vi "Oscilloscope_Dual_MohammadVersion.vi"() -> ()   [LabVIEW 2024]
uses:
  <vilib>/DAQmx/read.llb/DAQmx Read (Analog 1D Wfm NChan NSamp).vi
  <vilib>/DAQmx/create/channels.llb/DAQmx Create Channel (AI-Voltage-Basic).vi
  <vilib>/DAQmx/configure/timing.llb/DAQmx Timing (Sample Clock).vi
  <vilib>/DAQmx/configure/trigger.llb/DAQmx Start Trigger (Analog Edge).vi
  <vilib>/DAQmx/miscellaneous.llb/DAQmx Fill In Error Info.vi
panel:
  in  "stop":bool
  in  "Trigger source":string
  in  "File Logging":bool
  in  "Trigger Mode":bool
  in  "level":dbl format="%0.2f"
  out "right 2":dynamicdata(graph)=[{"t0"=timestamp(3806599236.6321588 s since 1904-01-01), "dt"=4.999999999999579e-07, "Y"=array[202167 elements], "attributes"=variant("NI_ChannelName"=variant(string "cDAQ2Mod1/ai1"), "NI_UnitDescription"=variant(string "Volts"))}]
  out "left 2":dynamicdata(graph)=[{"t0"=timestamp(3806599236.6321588 s since 1904-01-01), "dt"=4.999999999999579e-07, "Y"=array[202167 elements], "attributes"=variant("NI_ChannelName"=variant(string "cDAQ2Mod1/ai0"), "NI_UnitDescription"=variant(string "Volts"))}]
  in  "stop Acquisition":bool
  in  "File Name":string
  in  "Folder to save file to":path=path "A:/Source Localization/Material Evaluation paper/Dataset/Microphone Characterization/Clean Source"
  in  "physical channels":tag="cDAQ2Mod1/ai0, cDAQ2Mod1/ai3"
  in  "Sample Rate":dbl=200000.0 format="%0.2f"
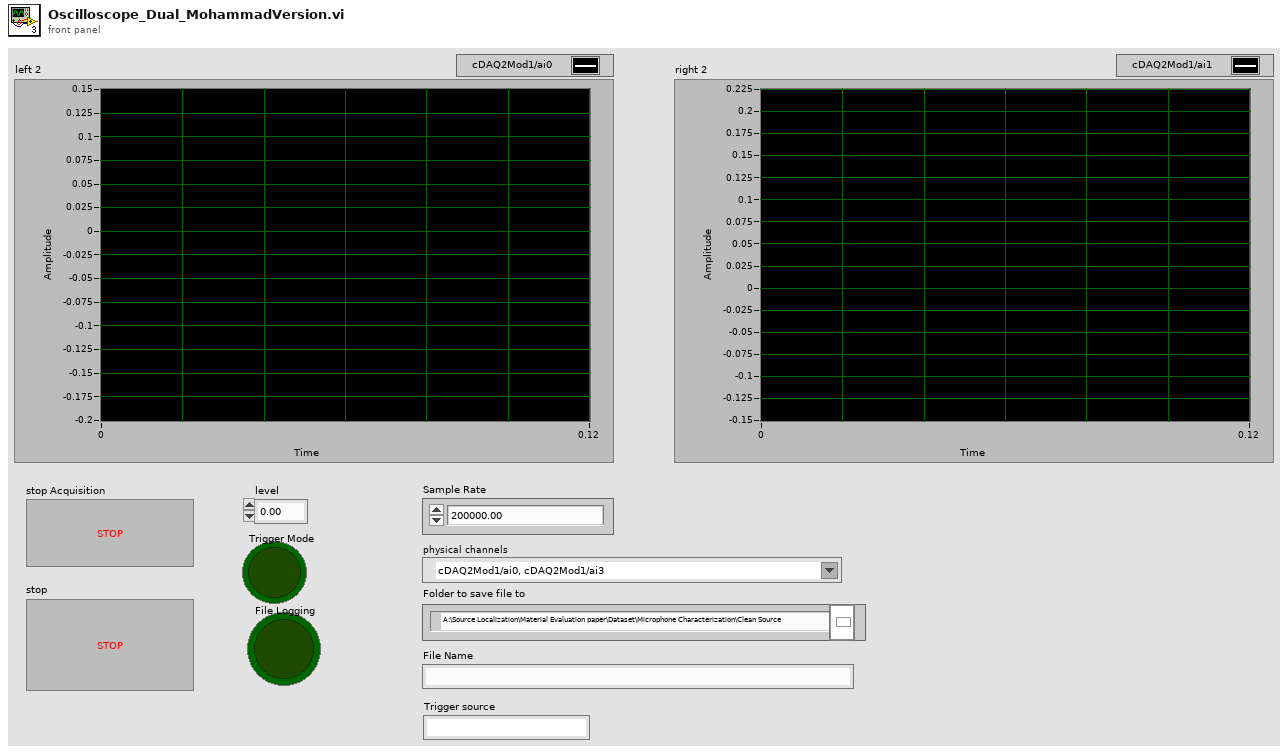
[diagram p1: front panel]
types:
  T1 = enum16{"open", "open or create", "create or replace", "create", "open (read-only)"}
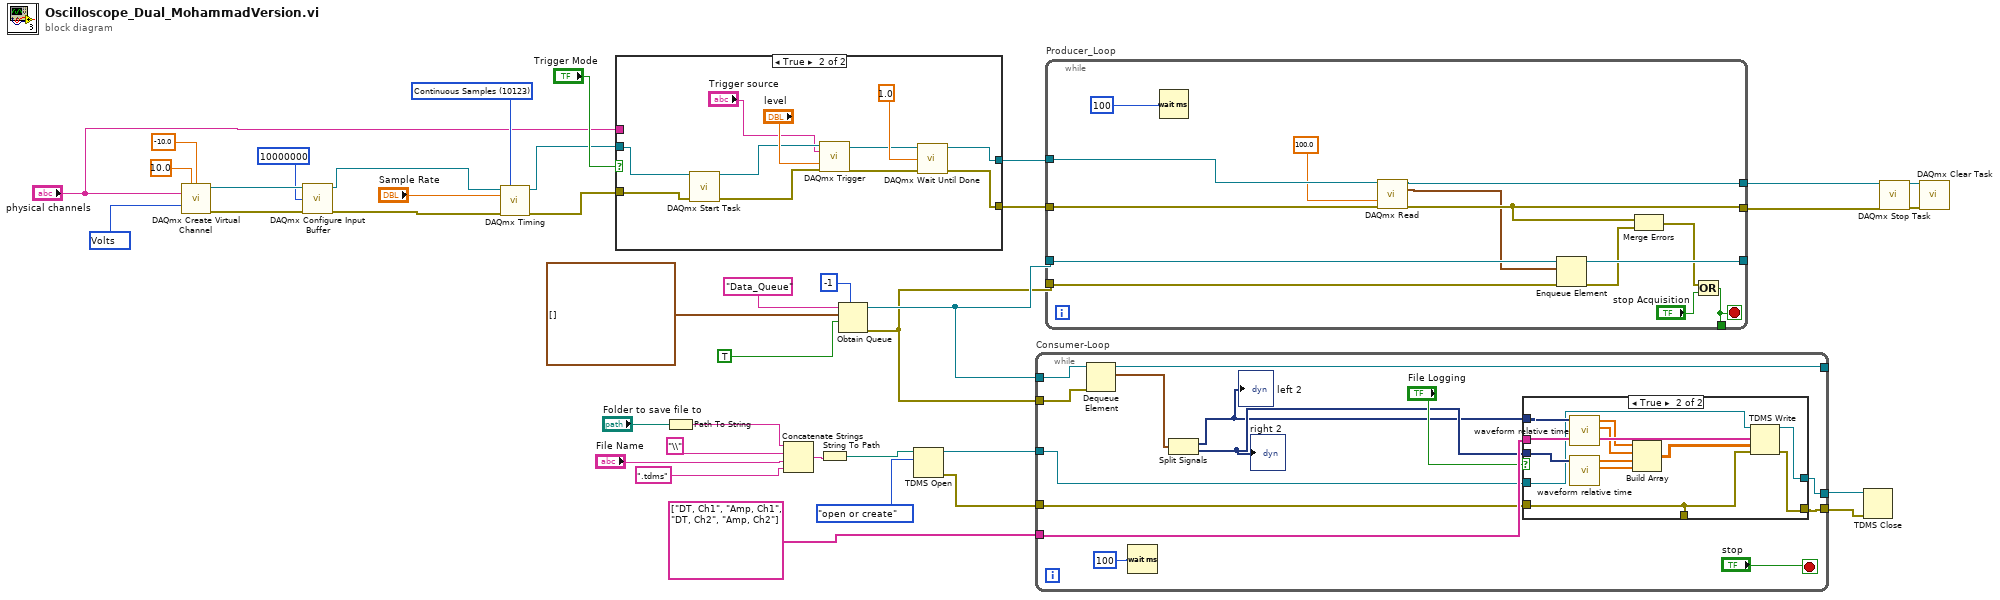
[diagram p0: block diagram]
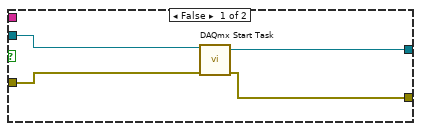
[diagram p2: hidden frame]
diagram:
  w10 = 10348 items=["Volts"=10348, "From Custom Scale"=10065] ("units")
  w34 = 10123 items=["Finite Samples"=10178, "Continuous Samples"=10123, "Hardware Timed Single Point"=12522] ("sample mode")
  n1 = call-poly <vilib>:"DAQmx Create Virtual Channel.vi"("maximum value"=10.0, "minimum value"=-10.0, "physical channels"="physical channels", "units"=w10) -> ("task out"=w39:refnum<k21>, "error out"=w38:errorcluster)  [unwired: 10 in]
  n2 = call <vilib>:"DAQmx Configure Input Buffer.vi"("task/channels in"=w39, "buffer size (in samples per channel)"=u32 10000000, "error in"=w38) -> ("task out"=w36:refnum<k21>, "error out"=w35:errorcluster)  [unwired: 11 in]
  n3 = call-poly <vilib>:"DAQmx Timing.vi"("task/channels in"=w36, "sample mode"=w34, "rate"="Sample Rate", "error in"=w35) -> ("task out"=w7:refnum<k21>, "error out"=w8:errorcluster)  [unwired: 10 in]
  n4 = case shown="True" "Trigger Mode" {
    tunnel: w8 -> [w41 w45]
    tunnel: w7 -> [w42 w46]
    tunnel: [w43 w50] -> w4
    tunnel: [w40 w49] -> w3
    tunnel: "physical channels" -> [_ _]
    frame False {
      n5 = call <vilib>:"DAQmx Start Task.vi"("task/channels in"=w42, "error in"=w41) -> ("task out"=w43:refnum<k21>, "error out"=w40:errorcluster)  [unwired: 12 in]
    }
    frame True {
      n6 = call <vilib>:"DAQmx Start Task.vi"("task/channels in"=w46, "error in"=w45) -> ("task out"=w48:refnum<k21>, "error out"=w47:errorcluster)  [unwired: 12 in]
      n7 = call-poly <vilib>:"DAQmx Trigger.vi"("task/channels in"=w48, "source"="Trigger source", "level"="level", "error in"=w47) -> ("task out"=w52:refnum<k21>, "error out"=w51:errorcluster)  [unwired: 10 in]
      n8 = call <vilib>:"DAQmx Wait Until Done.vi"("task/channels in"=w52, "timeout (sec)"=1.0, "error in"=w51) -> ("task out"=w50:refnum<k21>, "error out"=w49:errorcluster)  [unwired: 11 in]
    }
  }
  n9 = Path To String(path="Folder to save file to") -> (string=w29:string)
  n10 = Concatenate Strings(w29, "\\" ("string"), "File Name", ".tdms" ("string")) -> (w28:string)
  n11 = String To Path(string=w28) -> (path=w25:path)
  n12 = Obtain Queue(max queue size (-1, unlimited)=-1, name (unnamed)="Data_Queue", element data type=waveform(dbl)[] [] ("waveform"), create if not found? (T)=TRUE) -> (queue out=w19:refnum<queue>, error out=w15:errorcluster)  [unwired: 1 in, 1 out]
  n13 = TDMS Open(10:T1."open or create" ("operation (0:open)"), 11:w25) -> (0:w18:errorcluster, 3:w1:refnum<k34>)  [unwired: 5 in]
  n14 = while "Consumer-Loop" {
    tunnel: w19 -> [w68]
    tunnel: w18 -> [w62]
    tunnel: w15 -> [w67]
    tunnel: [w66] -> _
    tunnel: string[] ["DT, Ch1", "Amp, Ch1", "DT, Ch2", "Amp, Ch2"] ("channel name(s) in (Untitled)") -> [w65]
    tunnel: [w63] -> w13
    tunnel: [w61] -> w5
    tunnel: w1 -> [w57]
    stop <- "stop" stop-if-true
    n15 = Dequeue Element(queue=w68, error in (no error)=w67) -> (queue out=w66:refnum<queue>, element=w64:waveform(dbl)[])  [unwired: 1 in, 2 out]
    n16 = Wait (ms)(milliseconds to wait=u32 100) -> ()  [unwired: 1 out]
    n17 = Split Signals(w64) -> (w58:dynamicdata, w59:dynamicdata)  [unwired: 2 in]
    "left 2" <- w58
    "right 2" <- w59
    n18 = case shown="True" "File Logging" {
      tunnel: w65 -> [_ w82]
      tunnel: [w69 w81] -> w63
      tunnel: w62 -> [w70 w80]
      tunnel: [w70 w80] -> _
      tunnel: [w70 w79] -> w61
      tunnel: w59 -> [_ w74]
      tunnel: w58 -> [_ w73]
      tunnel: w57 -> [w69 w71]
      frame False {
      }
      frame True {
        n19 = call "waveform relative time.vi"("signal in"=w73) -> ("Y"=w78:dbl[], "Relative Time"=w77:dbl[])  [unwired: 7 in, 2 out]
        n20 = call "waveform relative time.vi"("signal in"=w74) -> ("Y"=w75:dbl[], "Relative Time"=w76:dbl[])  [unwired: 7 in, 2 out]
        n21 = Build Array(w77, w78, w76, w75) -> (w72:dbl[][])
        n22 = TDMS Write(0:w71, 7:w82, 9:w72, 11:w80) -> (4:w81:refnum<k34>, 15:w79:errorcluster)  [unwired: 2 in, 2 out]
      }
    }
  }
  n23 = while "Producer_Loop" {
    tunnel: w4 -> [w94]
    tunnel: w3 -> [w93]
    tunnel: w19 -> [w96]
    tunnel: w15 -> [w95]
    tunnel: [w92] -> _
    tunnel: [w88] -> w17
    tunnel: [w87] -> w16
    tunnel: [w83] -> _
    stop <- w83 stop-if-true
    n24 = Wait (ms)(milliseconds to wait=u32 100) -> ()  [unwired: 1 out]
    n25 = call-poly <vilib>:"DAQmx Read.vi"("task/channels in"=w94, "timeout"=100.0, "error in"=w93) -> ("task out"=w88:refnum<k21>, "data"=w86:waveform(dbl)[], "error out"=w87:errorcluster)  [unwired: 10 in]
    n26 = Enqueue Element(queue=w96, element=w86, error in (no error)=w95) -> (queue out=w92:refnum<queue>, error out=w91:errorcluster)  [unwired: 1 in, 1 out]
    n27 = Merge Errors(w87, w91) -> (w90:errorcluster)
    n28 = Or(x=w90, y="stop Acquisition") -> (x .or. y?=w83:bool)
  }
  n29 = TDMS Close(8:w5, 11:w13) -> ()  [unwired: 2 out]
  n30 = call <vilib>:"DAQmx Stop Task.vi"("task/channels in"=w17, "error in"=w16) -> ("task out"=w24:refnum<k21>, "error out"=w23:errorcluster)  [unwired: 12 in]
  n31 = call <vilib>:"DAQmx Clear Task.vi"("task in"=w24, "error in"=w23) -> ()  [unwired: 13 in, 1 out]
